vi "Actor Core.vi"(8 "error in":errorcluster, 11 "Actor_Autotest in":refnum<class "Actor_Autotest.lvclass">) -> (0 "error out":errorcluster, 3 "Actor out":refnum<class "Actor.lvclass">)   [LabVIEW 2020, in "Library Core.lvlib" / "Actor_Autotest.lvlib" / "Actor_Autotest.lvclass"]
doc: "(<B>Filename</B>: Actor Framework.lvlib:Actor.lvclass:Actor Core.vi)\n\nReceives messages to the actor, reacts to them, and initiates any error handling that may shut the actor down.\n\nDescendant classes may override this VI to append parallel tasks for the actor to complete while it handles messages. Overrides use the Call Parent Method node."
uses:
  Actor_Autotest.lvclass
  C:/Program Files (x86)/National Instruments/LabVIEW 2020/vi.lib/ActorFramework/Actor/Actor.lvclass
  <vilib>/ActorFramework/Actor/Actor.lvclass
  Actor_Autotest.lvclass/Actor_Autotest.ctl
  <vilib>/ActorFramework/Actor/Actor.lvclass/Actor.ctl
  <vilib>/ActorFramework/Message Enqueuer/Message Enqueuer.lvclass/Message Enqueuer.ctl
  Actor_Autotest Messages/Compute_Result Msg/Compute_Result Msg.lvclass/Compute_Result Msg.ctl
  <vilib>/ActorFramework/Message Enqueuer/Init from Existing Queue.vi
  <vilib>/ActorFramework/Message Enqueuer/Enqueue.vi
  <vilib>/ActorFramework/Stop Msg/Stop Msg.lvclass
  C:/Program Files (x86)/National Instruments/LabVIEW 2020/vi.lib/ActorFramework/Message/Message.lvclass
  Actor_Autotest Messages/Compute_Result Msg/Compute_Result Msg.lvclass
  <vilib>/ActorFramework/Message Priority Queue/Priority Enqueue.vi
  <vilib>/ActorFramework/Message Enqueuer/Message Enqueuer.lvclass
  Instrument/Instrument (Default)/Class Instrument (Default).lvclass
  Commun VI/Library Commun.lvlib
panel:
  out "Autotest":bool
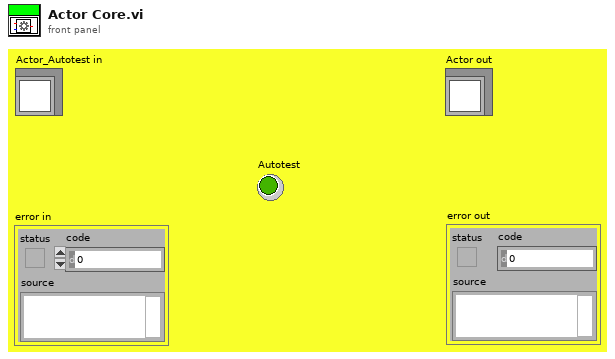
[diagram p1: front panel]
types:
  T1 = enum16{"Add Instr", "Remove Instr", "List Instr", "Get Instr Class", "Get Instr obj", "Save Insrt obj", "Modify Insrt obj", "Init"}
  T2 = cluster{"Name":string, "Instrument":refnum<class "Class Instrument (Default).lvclass">, "Close After Autotest":bool}
  T3 = cluster{"Name":string, "Instrument":refnum<class "Class Instrument (Default).lvclass">, "Close After Autotest":bool}[]
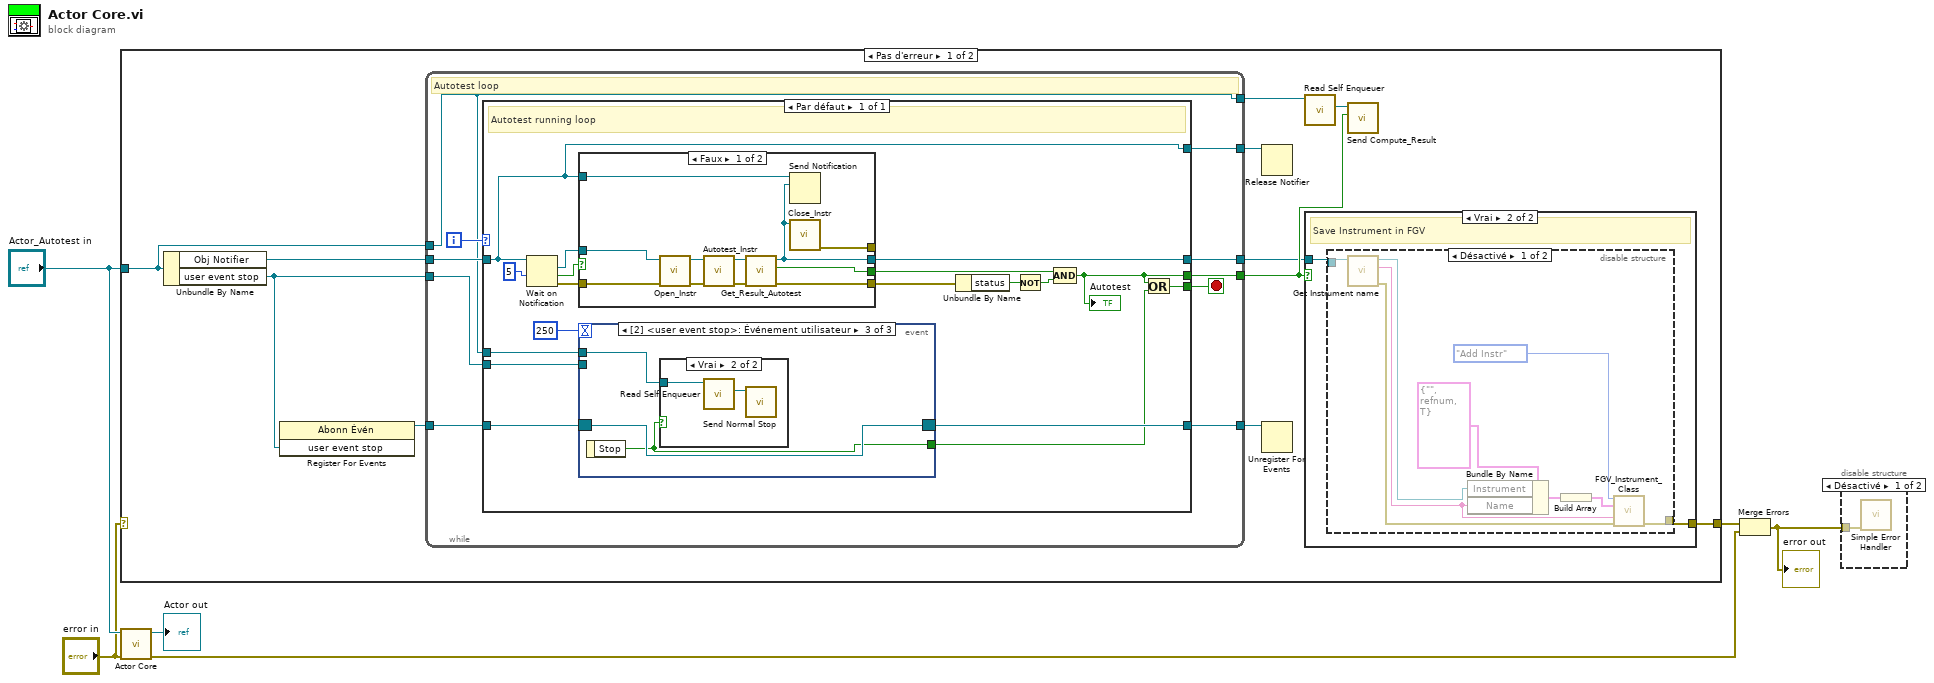
[diagram p0: block diagram]
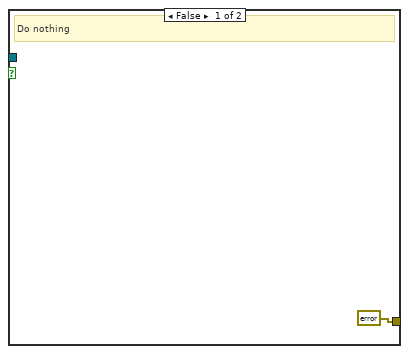
[diagram p3: hidden frame]
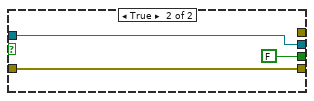
[diagram p5: hidden frame]
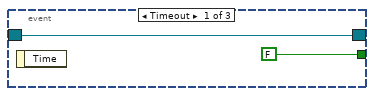
[diagram p6: hidden frame]
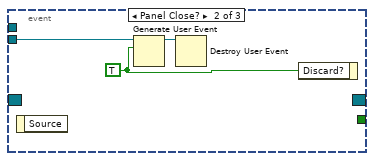
[diagram p7: hidden frame]
diagram:
  n1 = case shown="Pas d'erreur" "error in" {
    selector: "error in" -> [_ w82]
    tunnel: "Actor_Autotest in" -> [w14 _]
    tunnel: [w10 w82] -> w3
    frame No Error {
      n2 = Unbundle By Name(w14) -> ("Obj Notifier"=w15:refnum<notifier>, "user event stop"=w7:refnum<user-event>)
      n3 = register-events(w7) -> (reference out=w17:refnum<event-registration>)  [unwired: 2 in, 1 out]
      n4 = while {
        tunnel: w17 -> [w39]
        tunnel: [w38] -> w16
        tunnel: [w37] -> w11
        tunnel: w15 -> [w34]
        tunnel: w14 -> [w32]
        tunnel: [w32] -> w9
        tunnel: [w33] -> w12
        tunnel: [w31] -> w8
        tunnel: w7 -> [w30]
        i -> [w35]
        stop <- w36 stop-if-true
        # "Autotest loop"
        n5 = case shown="Par défaut" w35 {
          tunnel: w39 -> [w53]
          tunnel: [w52] -> w38
          tunnel: [w50] -> w37
          tunnel: [w49] -> w36
          tunnel: w34 -> [w41]
          tunnel: [w45] -> w33
          tunnel: w32 -> [w44]
          tunnel: [w41] -> w31
          tunnel: w30 -> [w40]
          frame Par défaut {
            # "Autotest running loop"
            n6 = Wait on Notification(notifier=w41, timeout in ms (-1)=5) -> (notification=w47:refnum<class "Class Instrument (Default).lvclass">, timed out?=w42:bool, error out=w48:errorcluster)  [unwired: 2 in, 1 out]
            n7 = case shown="Faux" w42 {
              tunnel: [w62 w71] -> w57
              tunnel: [w67 FALSE ("Autotest Ok ?")] -> w54
              tunnel: [w59 w70] -> w50
              tunnel: w48 -> [w66 w71]
              tunnel: w47 -> [w65 w70]
              tunnel: w41 -> [w63 _]
              tunnel: [w58 _] -> _
              frame False {
                n8 = call-dynamic "Open_Instr.vi"("error in (no error)"=w66, "Class Multimeter (Default) en entrée"=w65) -> ("error out"=w64:errorcluster, "Class Multimeter (Default) en sortie"=w68:refnum<class "Class Instrument (Default).lvclass">)  [unwired: 8 in]
                n9 = call-dynamic "Autotest_Instr.vi"("error in (no error)"=w64, "Class Instrument (Default) en entrée"=w68) -> ("error out"=w60:errorcluster, "Class Instrument (Default) en sortie"=w61:refnum<class "Class Instrument (Default).lvclass">)  [unwired: 8 in]
                n10 = call-dynamic "Get_Result_Autotest.vi"("error in (no error)"=w60, "Class Instrument (Default) en entrée"=w61) -> ("error out"=w62:errorcluster, "Autotest Ok ?"=w67:bool, "Class Instrument (Default) en sortie"=w59:refnum<class "Class Instrument (Default).lvclass">)  [unwired: 7 in]
                n11 = Send Notification(notification=w59, notifier=w63) -> ()  [unwired: 1 in, 2 out]
                n12 = call-dynamic "Close_Instr.vi"("Class Instrument (Default) en entrée"=w59) -> ("error out"=w58:errorcluster)  [unwired: 9 in, 1 out]
              }
              frame True {
              }
            }
            n13 = event shown="[2] <user event stop>: Événement utilisateur" {
              selector: w53 -> [w73 _ w79]
              dyn-events: [w73 _ w79] -> w52
              timeout: 250 -> [_ _ _]
              tunnel: [FALSE ("Stop") _ w78] -> w46
              tunnel: w44 -> [_ _ w77]
              tunnel: w40 -> [_ w74 _]
              event Timeout {
                n14 = event-data() -> ()  [unwired: 1 in, 1 out]
              }
              event Panel Close? {
                w75 = TRUE ("event data")
                n15 = event-data() -> ()  [unwired: 1 in, 1 out]
                n16 = Generate User Event(user event=w74, event data cluster=w75) -> (user event out=w76:refnum<user-event>)  [unwired: 2 in, 1 out]
                n17 = Destroy User Event(user event=w76) -> ()  [unwired: 1 in, 1 out]
                n18 = event-data("Discard?"=w75) -> ()  [unwired: 1 in, 1 out]
              }
              event User Event {
                n19 = event-data() -> ("Stop"=w78:bool)  [unwired: 1 in]
                n20 = case shown="Vrai" w78 {
                  tunnel: w77 -> [_ w81]
                  frame False {
                  }
                  frame True {
                    n21 = call <vilib>:"Read Self Enqueuer.vi"("Actor"=w81) -> ("Self Enqueuer"=w80:refnum<class "Message Enqueuer.lvclass">)  [unwired: 10 in]
                    n22 = call <vilib>:"Send Normal Stop.vi"("Message Enqueuer"=w80) -> ()  [unwired: 10 in, 1 out]
                  }
                }
              }
            }
            n23 = Unbundle By Name(w57) -> ("status"=w56:bool)
            n24 = Not(x=w56) -> (.not. x?=w55:bool)
            n25 = Compound Arithmetic op=AND(w54, w55) -> (w45:bool)
            "Autotest" <- w45
            n26 = Or(x=w45, y=w46) -> (x .or. y?=w49:bool)
          }
        }
      }
      n27 = Release Notifier(notifier=w8) -> ()  [unwired: 2 in, 3 out]
      n28 = Unregister For Events(event registration refnum=w16) -> ()  [unwired: 1 in, 1 out]
      n29 = call <vilib>:"Read Self Enqueuer.vi"("Actor"=w9) -> ("Self Enqueuer"=w13:refnum<class "Message Enqueuer.lvclass">)  [unwired: 10 in]
      n30 = case shown="Vrai" w12 {
        tunnel: w11 -> [_ w19]
        tunnel: [errorcluster {"status"=FALSE, "code"=0, "source"=""} ("error out") w20] -> w10
        frame False {
          # "Do nothing"
        }
        frame True {
          # "Save Instrument in FGV"
          n31 = disable-structure shown="Désactivé" {
            disable-tunnel: [w29 _] -> w20
            disable-tunnel: w19 -> [w28 _]
            frame Disabled {
              n32 = call-dynamic "Get Instrument name .vi"("Class Instrument (Default) en entrée"=w28) -> ("error out"=w27:errorcluster, "Instrument name"=w26:string, "Class Instrument (Default) en sortie"=w25:refnum<class "Class Instrument (Default).lvclass">)  [unwired: 8 in]
              n33 = Bundle By Name(cluster=T2 {"Name"="", "Instrument"=refnum, "Close After Autotest"=TRUE} ("Cluster"), "Instrument"=w25, "Name"=w26) -> (w24:T2)
              n34 = Build Array(w24) -> (w23:T3)
              n35 = call "FGV_Instrument_Class.vi"("Action"=T1."Add Instr", "Instruments"=w23, "Instr name"=w26, "error in (no error)"=w27) -> ("error out"=w29:errorcluster)  [unwired: 9 in, 2 out]
            }
            frame Enabled {
            }
          }
        }
      }
      n36 = call "Send Compute_Result.vi"("Autotest?"=w12, "Message Enqueuer"=w13) -> ()  [unwired: 8 in, 2 out]
    }
    frame Error {
    }
  }
  n37 = call-parent "Actor Core.vi"("error in"="error in", "Actor in"="Actor_Autotest in") -> ("error out"=w2:errorcluster, "Actor out"=→"Actor out":refnum<class "Actor.lvclass">)  [unwired: 8 in]
  n38 = Merge Errors(w3, w2) -> (w1:errorcluster)
  "error out" <- w1
  n39 = disable-structure shown="Désactivé" {
    disable-tunnel: w1 -> [w83 _]
    frame Disabled {
      n40 = call <vilib>:"Simple Error Handler.vi"("error in (no error)"=w83) -> ()  [unwired: 4 in, 5 out]
    }
    frame Enabled {
    }
  }
